vi "Calculate Timeout.vi"(8 "error in (no error)":errorcluster, 10 "relative seconds":dbl, 11 "timeout in ms (-1) in":i32) -> (0 "error out":errorcluster, 3 "timeout in ms (-1) out":i32)   [LabVIEW 2017, in "Promise Future.lvlib" / "Future.lvclass"]
uses:
  Future.lvclass
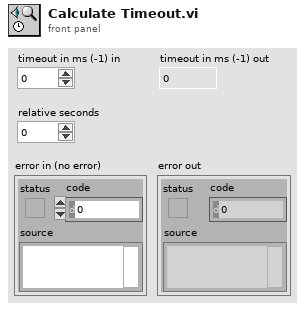
[diagram p1: front panel]
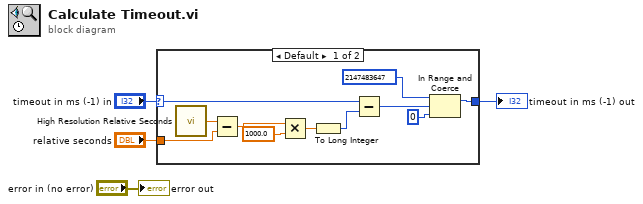
[diagram p0: block diagram]
diagram:
  n1 = case shown="Default" "timeout in ms (-1) in" {
    selector: "timeout in ms (-1) in" -> [w15 w16]
    tunnel: "relative seconds" -> [w13 _]
    tunnel: [w7 w16] -> w4
    frame Default {
      n2 = call <vilib>:"High Resolution Relative Seconds.vi"() -> ("relative seconds"=w14:dbl)
      n3 = Subtract(x=w14, y=w13) -> (x-y=w12:dbl)
      n4 = Multiply(x=w12, y=1000.0 ("x")) -> (x*y=w10:dbl)
      n5 = To Long Integer(number=w10) -> (32bit integer=w9:i32)
      n6 = Subtract(x=w15, y=w9) -> (x-y=w8:i32)
      n7 = In Range and Coerce(upper limit=2147483647, x=w8, lower limit=0) -> (coerced(x)=w7:i32)  [unwired: 1 out]
    }
    frame -1, 0 {
    }
  }
  "timeout in ms (-1) out" <- w4
  "error out" <- "error in (no error)"
